vi "Search Cache.vi"(8 "error in":errorcluster, 10 "SNAME":string, 11 "ParseGDSII in":refnum<class "ParseGDSII.lvclass">) -> (0 "error out":errorcluster, 1 "Found":bool, 2 "Index":i32, 3 "ParseGDSII out":refnum<class "ParseGDSII.lvclass">)   [LabVIEW 2019, in "ParseGDSII.lvclass"]
uses:
  ParseGDSII.lvclass
  ParseGDSII.lvclass/ParseGDSII.ctl
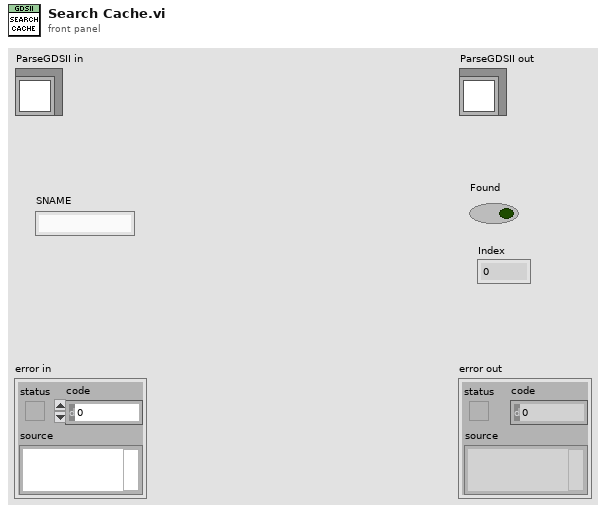
[diagram p1: front panel]
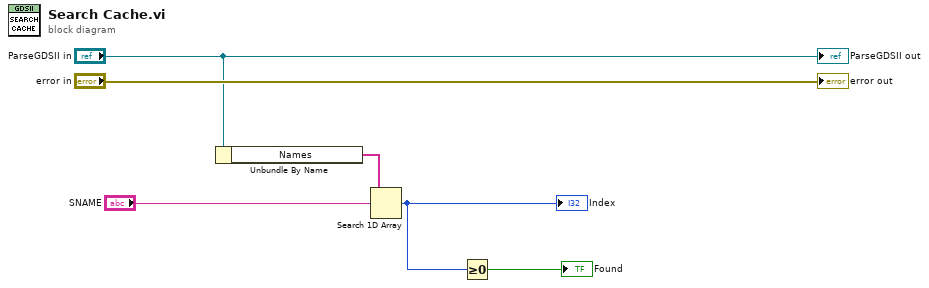
[diagram p0: block diagram]
diagram:
  n1 = Unbundle By Name("ParseGDSII in") -> ("Names"=w1:string[])
  n2 = Search 1D Array(1D array=w1, element="SNAME") -> (index of element=w5:i32)  [unwired: 1 in]
  "Index" <- w5
  n3 = Greater Or Equal To 0?(x=w5) -> (x >= 0?=→"Found":bool)
  "error out" <- "error in"
  "ParseGDSII out" <- "ParseGDSII in"
